vi "JV Data analysis from master log file.vi"(9 "Experiment Indicator":string, 11 "Master log filepath":path) -> ()   [LabVIEW 2011]
panel:
  out "Array":string[](array[string])
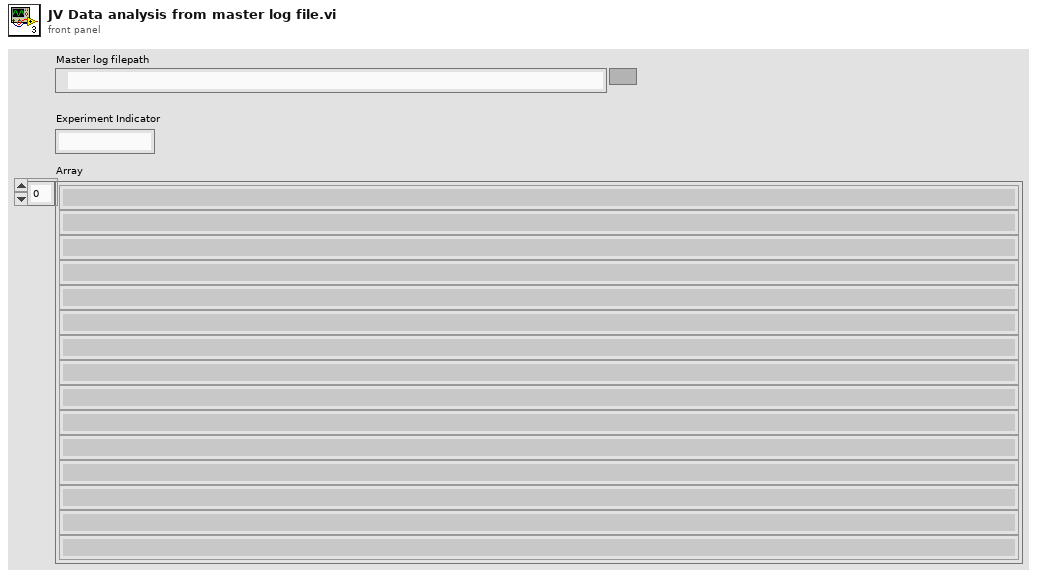
[diagram p1: front panel]
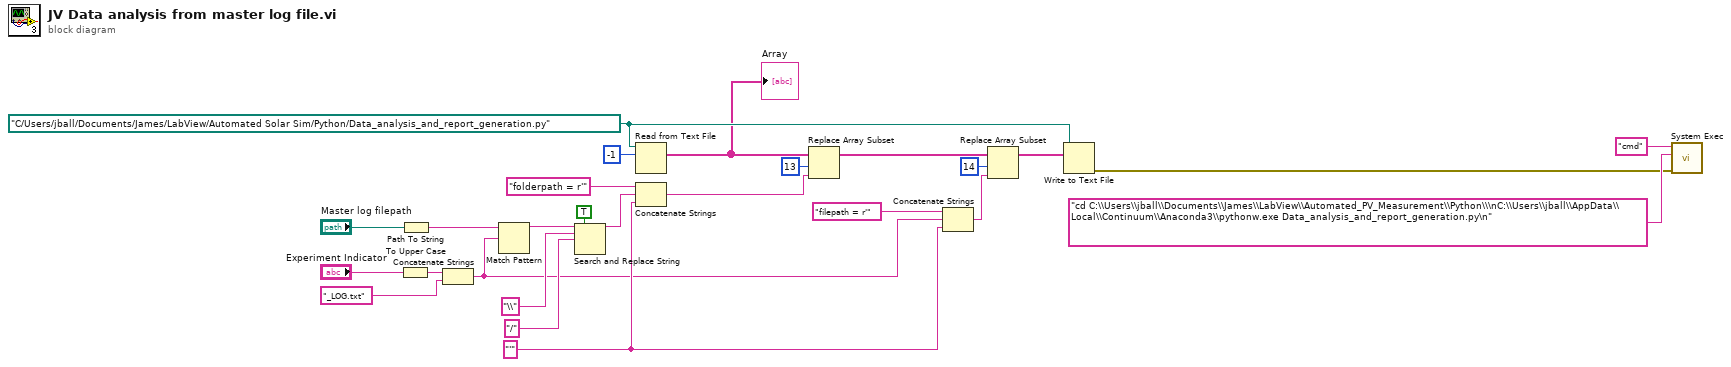
[diagram p0: block diagram]
diagram:
  w11 = "'" ("string")
  w16 = path "C:/Users/jball/Documents/James/LabView/Automated Solar Sim/Python/Data_analysis_and_report_generation.py" ("file (use dialog)")
  n1 = To Upper Case(1:"Experiment Indicator") -> (0:w10:string)
  n2 = Path To String(path="Master log filepath") -> (string=w5:string)
  n3 = Concatenate Strings(w10, "_LOG.txt") -> (w6:string)
  n4 = Match Pattern(string=w5, regular expression=w6) -> (before substring=w4:string)  [unwired: 1 in, 3 out]
  n5 = Search and Replace String(replace all?=TRUE ("replace all? (F)"), input string=w4, search string="\\", replace string="/" ("search string")) -> (result string=w3:string)  [unwired: 4 in, 3 out]
  n6 = Read from Text File(file (use dialog)=w16, count=-1) -> (text=w1:string[])  [unwired: 2 in, 3 out]
  "Array" <- w1
  n7 = Concatenate Strings("folderpath = r'" ("string"), w3, w11) -> (w20:string)
  n8 = Replace Array Subset(array=w1, new element=w20, index=13) -> (w22:string[])
  n9 = Concatenate Strings("filepath = r'" ("string"), w6, w11) -> (w18:string)
  n10 = Replace Array Subset(array=w22, new element=w18, index=14) -> (w15:string[])
  n11 = Write to Text File(file (use dialog)=w16, text=w15) -> (error out=w17:errorcluster)  [unwired: 2 in, 2 out]
  n12 = call <vilib>:"System Exec.vi"("error in (no error)"=w17, "standard input"="cd C:\\Users\\jball\\Documents\\James\\LabView\\Automated_PV_Measurement\\Python\\\nC:\\Users\\jball\\AppData\\Local\\Continuum\\Anaconda3\\pythonw.exe Data_analysis_and_report_generation.py\n", "command line"="cmd") -> ()  [unwired: 5 in, 4 out]
